vi "Swerve Math.vi"(0 "Gyro":dbl, 1 "FWD":dbl(slide) scale=-1.0..1.0, 2 "STR":dbl(slide) scale=-1.0..1.0, 3 "RCW":dbl(slide) scale=-1.0..1.0) -> (7 "Wheel Speeds":dbl[](array[numeric]), 9 "Wheel Angles":dbl[](array[numeric]))   [LabVIEW 2023]
uses:
  Framework/Robot Global Data.vi
panel:
  in  "Gyro Working":bool=TRUE
  out "STR(Field)":dbl
  out "FWD(Field)":dbl
  out "MAX(before normalized)":dbl
  out "WA 4":dbl
  out "WA 3":dbl
  out "WA 2":dbl
  out "WA 1":dbl
  out "WS 4":dbl
  out "WS 3":dbl
  out "WS 2":dbl
  out "WS 1":dbl
  out "D":dbl
  out "C":dbl
  out "B":dbl
  out "A":dbl
  in  "Width(Left to Right)":dbl=20.0
  in  "Length(Front to Back)":dbl=28.0
  # "From the Center of the Wheels"
  # "Forward/Back"
  # "Left/Right"
  # "Rotation(Clockwise)"
  # "Units are irrelevant"
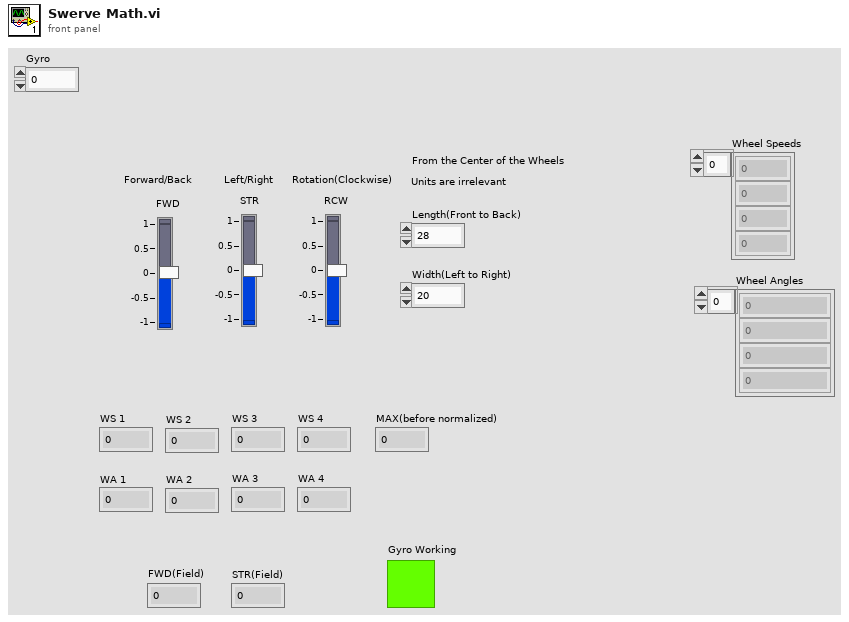
[diagram p1: front panel]
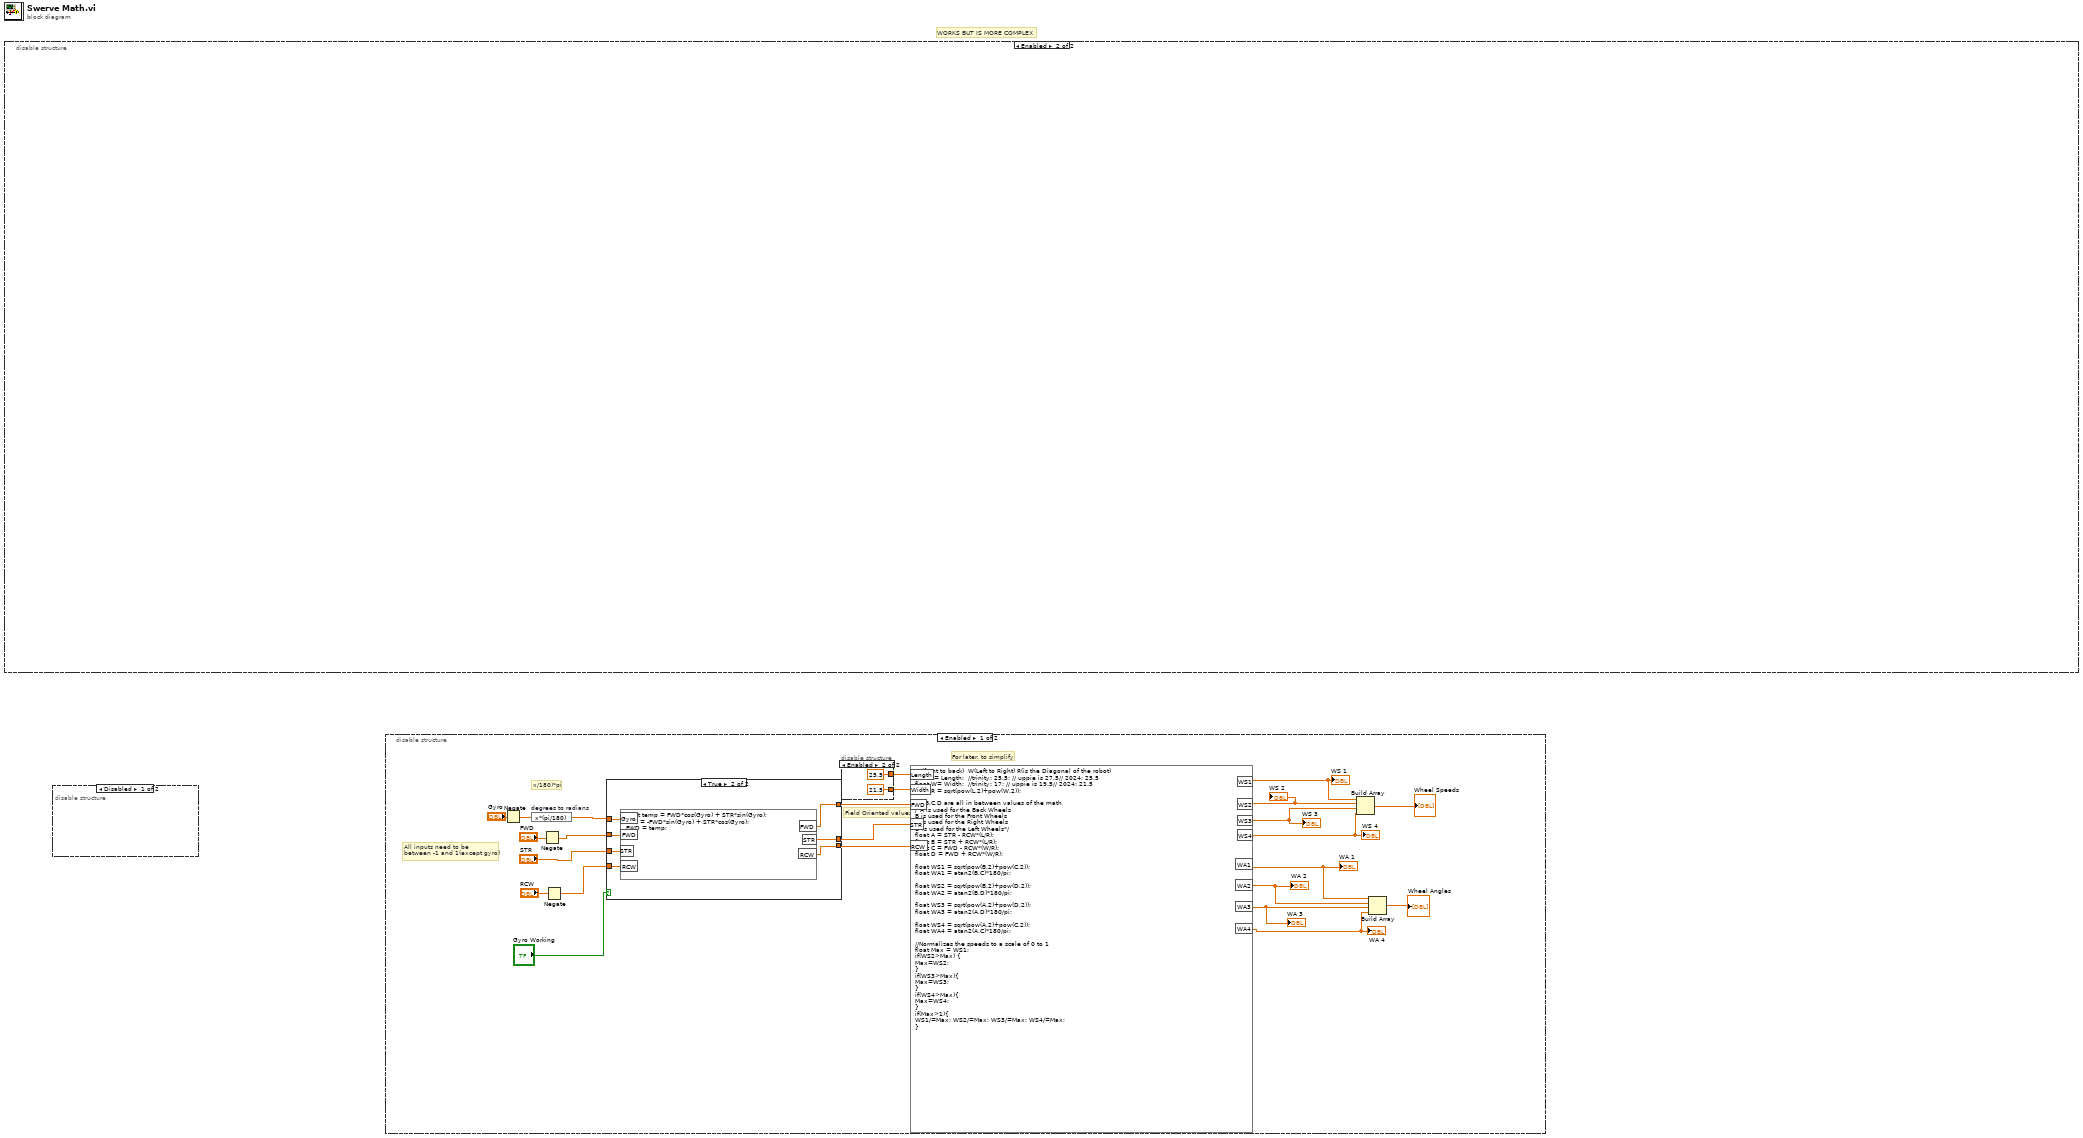
[diagram p0: block diagram]
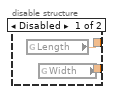
[diagram p3: hidden frame]
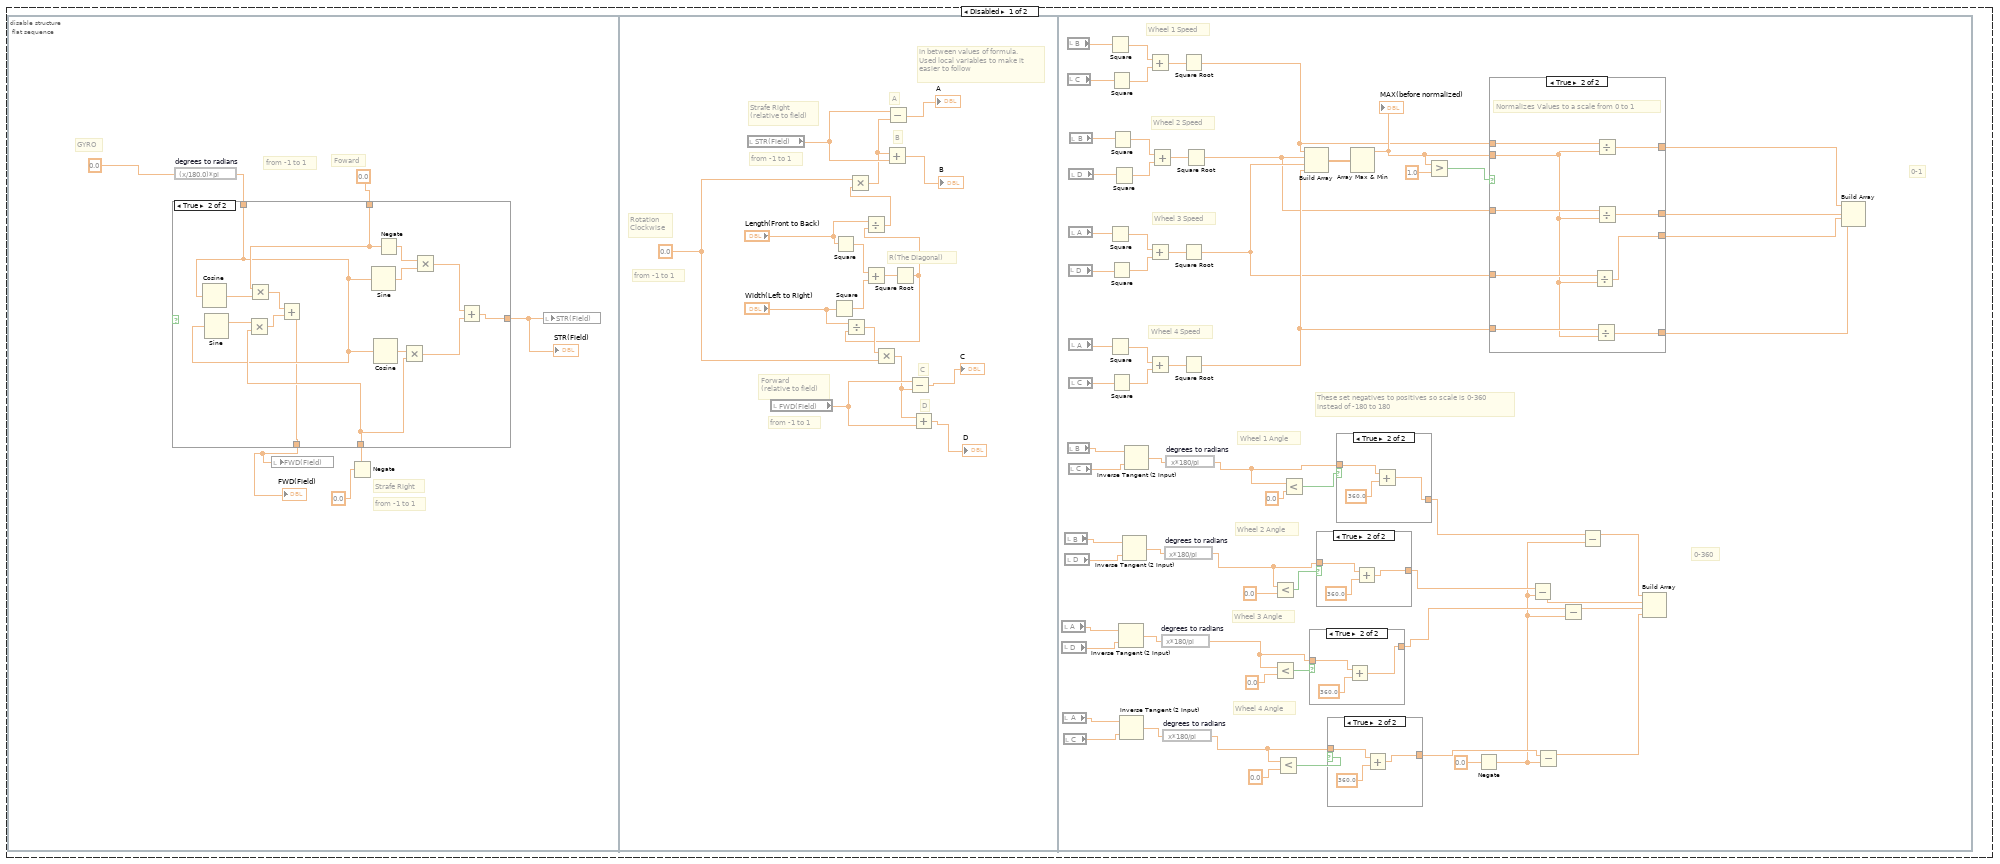
[diagram p6: hidden frame]
diagram:
  # "WORKS BUT IS MORE COMPLEX"
  n1 = disable-structure shown="Enabled" {
    frame Disabled {
      n2 = flat-sequence {
        frame #0 {
          # "GYRO"
          # "from -1 to 1"
          # "from -1 to 1"
          # "Strafe Right"
          # "Foward"
          n3 = expression code="(x/180.0)*pi" "degrees to radians"(0.0) -> (w5:dbl)
          n4 = Negate(x=0.0) -> (-x=w4:dbl)
          n5 = case shown="True" {
            selector: _ -> [_ _]
            tunnel: w4 -> [w9 w14]
            tunnel: 0.0 ("FWD") -> [w8 w13]
            tunnel: [w9 w12] -> w7
            tunnel: w5 -> [_ w11]
            tunnel: [w8 w10] -> w6
            frame False {
            }
            frame True {
              n6 = Cosine(x=w11) -> (cos(x)=w15:dbl)
              n7 = Sine(x=w11) -> (sin(x)=w16:dbl)
              n8 = Multiply(x=w16, y=w14) -> (x*y=w17:dbl)
              n9 = Multiply(x=w13, y=w15) -> (x*y=w18:dbl)
              n10 = Add(x=w18, y=w17) -> (x+y=w10:dbl)
              n11 = Sine(x=w11) -> (sin(x)=w23:dbl)
              n12 = Cosine(x=w11) -> (cos(x)=w22:dbl)
              n13 = Negate(x=w13) -> (-x=w21:dbl)
              n14 = Multiply(x=w22, y=w14) -> (x*y=w20:dbl)
              n15 = Multiply(x=w21, y=w23) -> (x*y=w19:dbl)
              n16 = Add(x=w19, y=w20) -> (x+y=w12:dbl)
            }
          }
          "STR(Field)" <- w7
          "FWD(Field)" <- w6
          n17 = local write "FWD(Field)"(w6) -> ()
          n18 = local write "STR(Field)"(w7) -> ()
        }
        frame #1 {
          w24 = 0.0 ("x")
          # "from -1 to 1"
          # "from -1 to 1"
          # "from -1 to 1"
          # "in between values of formula.\nUsed local variables to make it\neasier to follow"
          # "Rotation\nClockwise"
          # "Forward\n(relative to field)"
          # "Strafe Right\n(relative to field)"
          # "D"
          # "C"
          # "B"
          # "A"
          # "R(The Diagonal)"
          n19 = local read "STR(Field)"() -> (w40:dbl)
          n20 = local read "FWD(Field)"() -> (w39:dbl)
          n21 = Square(x="Width(Left to Right)") -> (x^2=w27:dbl)
          n22 = Square(x="Length(Front to Back)") -> (x^2=w26:dbl)
          n23 = Add(x=w26, y=w27) -> (x+y=w25:dbl)
          n24 = Square Root(x=w25) -> (sqrt(x)=w29:dbl)
          n25 = Divide(x="Width(Left to Right)", y=w29) -> (x/y=w32:dbl)
          n26 = Divide(x="Length(Front to Back)", y=w29) -> (x/y=w31:dbl)
          n27 = Multiply(x=w24, y=w31) -> (x*y=w33:dbl)
          n28 = Multiply(x=w32, y=w24) -> (x*y=w34:dbl)
          n29 = Add(x=w33, y=w40) -> (x+y=→"B":dbl)
          n30 = Subtract(x=w40, y=w33) -> (x-y=→"A":dbl)
          n31 = Subtract(x=w39, y=w34) -> (x-y=→"C":dbl)
          n32 = Add(x=w34, y=w39) -> (x+y=→"D":dbl)
        }
        frame #2 {
          # "0-360"
          # "0-1"
          # "These set negatives to positives so scale is 0-360\ninstead of -180 to 180"
          # "Wheel 4 Angle"
          # "Wheel 3 Angle"
          # "Wheel 2 Angle"
          # "Wheel 1 Angle"
          # "Wheel 4 Speed"
          # "Wheel 3 Speed"
          # "Wheel 2 Speed"
          # "Wheel 1 Speed"
          n33 = local read "A"() -> (w82:dbl)
          n34 = local read "D"() -> (w83:dbl)
          n35 = local read "A"() -> (w84:dbl)
          n36 = local read "C"() -> (w85:dbl)
          n37 = local read "B"() -> (w80:dbl)
          n38 = local read "D"() -> (w81:dbl)
          n39 = local read "B"() -> (w57:dbl)
          n40 = local read "C"() -> (w56:dbl)
          n41 = local read "B"() -> (w78:dbl)
          n42 = local read "D"() -> (w67:dbl)
          n43 = local read "C"() -> (w79:dbl)
          n44 = local read "D"() -> (w61:dbl)
          n45 = local read "A"() -> (w66:dbl)
          n46 = local read "A"() -> (w71:dbl)
          n47 = local read "C"() -> (w72:dbl)
          n48 = local read "B"() -> (w62:dbl)
          n49 = Square(x=w57) -> (x^2=w55:dbl)
          n50 = Square(x=w66) -> (x^2=w65:dbl)
          n51 = Square(x=w71) -> (x^2=w70:dbl)
          n52 = Square(x=w56) -> (x^2=w54:dbl)
          n53 = Square(x=w67) -> (x^2=w64:dbl)
          n54 = Square(x=w72) -> (x^2=w69:dbl)
          n55 = Square(x=w62) -> (x^2=w60:dbl)
          n56 = Square(x=w61) -> (x^2=w59:dbl)
          n57 = Inverse Tangent (2 Input)(1:w83, 2:w82) -> (0:w100:dbl)
          n58 = Inverse Tangent (2 Input)(1:w85, 2:w84) -> (0:w102:dbl)
          n59 = Inverse Tangent (2 Input)(1:w81, 2:w80) -> (0:w98:dbl)
          n60 = Inverse Tangent (2 Input)(1:w79, 2:w78) -> (0:w96:dbl)
          n61 = Add(x=w55, y=w54) -> (x+y=w53:dbl)
          n62 = Add(x=w65, y=w64) -> (x+y=w63:dbl)
          n63 = Add(x=w70, y=w69) -> (x+y=w68:dbl)
          n64 = Add(x=w60, y=w59) -> (x+y=w58:dbl)
          n65 = expression code="x*180/pi" "degrees to radians"(w100) -> (w101:dbl)
          n66 = expression code="x*180/pi" "degrees to radians"(w102) -> (w103:dbl)
          n67 = expression code="x*180/pi" "degrees to radians"(w98) -> (w99:dbl)
          n68 = expression code="x*180/pi" "degrees to radians"(w96) -> (w97:dbl)
          n69 = Square Root(x=w53) -> (sqrt(x)=w75:dbl)
          n70 = Square Root(x=w63) -> (sqrt(x)=w76:dbl)
          n71 = Square Root(x=w68) -> (sqrt(x)=w77:dbl)
          n72 = Square Root(x=w58) -> (sqrt(x)=w74:dbl)
          n73 = Less?(x=w99, y=0.0) -> (x < y?=w89:bool)
          n74 = Less?(x=w101, y=0.0) -> (x < y?=w88:bool)
          n75 = Less?(x=w103, y=0.0) -> (x < y?=w87:bool)
          n76 = Less?(x=w97, y=0.0) -> (x < y?=w86:bool)
          n77 = Build Array(w75, w74, w76, w77) -> (w73:dbl[])
          n78 = case shown="True" w88 {
            tunnel: w101 -> [w124 w126]
            tunnel: [w124 w125] -> w105
            frame False {
            }
            frame True {
              n79 = Add(x=w126, y=360.0) -> (x+y=w125:dbl)
            }
          }
          n80 = case shown="True" w89 {
            tunnel: w99 -> [w120 w122]
            tunnel: [w120 w121] -> w104
            frame False {
            }
            frame True {
              n81 = Add(x=w122, y=360.0) -> (x+y=w121:dbl)
            }
          }
          n82 = case shown="True" w87 {
            tunnel: w103 -> [w128 w130]
            tunnel: [w128 w129] -> w106
            frame False {
            }
            frame True {
              n83 = Add(x=w130, y=360.0) -> (x+y=w129:dbl)
            }
          }
          n84 = case shown="True" w86 {
            tunnel: w97 -> [w132 w134]
            tunnel: [w132 w133] -> w44
            frame False {
            }
            frame True {
              n85 = Add(x=w134, y=360.0) -> (x+y=w133:dbl)
            }
          }
          n86 = Array Max & Min(array=w73) -> (max value=w90:dbl)  [unwired: 3 out]
          "MAX(before normalized)" <- w90
          n87 = Greater?(x=w90, y=1.0) -> (0:w91:bool)
          n88 = Negate(x=0.0) -> (-x=w45:dbl)
          n89 = case shown="True" w91 {
            tunnel: w74 -> [w109 w119]
            tunnel: w75 -> [w110 w118]
            tunnel: w76 -> [w108 w117]
            tunnel: w77 -> [w107 w116]
            tunnel: w90 -> [_ w115]
            tunnel: [w110 w114] -> w92
            tunnel: [w109 w113] -> w93
            tunnel: [w108 w112] -> w94
            tunnel: [w107 w111] -> w95
            frame False {
            }
            frame True {
              # "Normalizes Values to a scale from 0 to 1"
              n90 = Divide(x=w117, y=w115) -> (x/y=w112:dbl)
              n91 = Divide(x=w116, y=w115) -> (x/y=w111:dbl)
              n92 = Divide(x=w118, y=w115) -> (x/y=w114:dbl)
              n93 = Divide(x=w119, y=w115) -> (x/y=w113:dbl)
            }
          }
          n94 = Subtract(x=w104, y=w45) -> (x-y=w42:dbl)
          n95 = Subtract(x=w106, y=w45) -> (x-y=w46:dbl)
          n96 = Subtract(x=w105, y=w45) -> (x-y=w43:dbl)
          n97 = Subtract(x=w44, y=w45) -> (x-y=w47:dbl)
          n98 = Build Array(w47, w42, w43, w46) -> ()  [unwired: 1 out]
          n99 = Build Array(w92, w93, w94, w95) -> ()  [unwired: 1 out]
        }
      }
    }
    frame Enabled {
    }
  }
  n100 = disable-structure shown="Disabled" {
    frame Disabled {
    }
    frame Enabled {
    }
  }
  n101 = disable-structure shown="Enabled" {
    frame Enabled {
      # "x/180)*pi"
      # "Field Oriented values"
      # "All inputs need to be\nbetween -1 and 1(except gyro)"
      # "For later, to simplify"
      n102 = Negate(x="Gyro") -> (-x=w136:dbl)
      n103 = expression code="x*(pi/180)" "degrees to radians"(w136) -> (w155:dbl)
      n104 = Negate(x="FWD") -> (-x=w142:dbl)
      n105 = Negate(x="RCW") -> (-x=w140:dbl)
      n106 = case shown="True" "Gyro Working" {
        tunnel: [w166 w173] -> w158
        tunnel: [w165 w172] -> w157
        tunnel: [w164 w171] -> w156
        tunnel: w155 -> [_ w170]
        tunnel: w142 -> [w166 w169]
        tunnel: w140 -> [w164 w168]
        tunnel: "STR" -> [w165 w167]
        frame False {
        }
        frame True {
          n107 = formula code="float temp = FWD*cos(Gyro) + STR*sin(Gyro); \nSTR = -FWD*sin(Gyro) + STR*cos(Gyro); \nFWD = temp;"("Gyro"=w170, "FWD"=w169, "STR"=w167, "RCW"=w168) -> ("FWD"=w173:dbl, "STR"=w172:dbl, "RCW"=w171:dbl)
        }
      }
      n108 = disable-structure shown="Enabled" {
        disable-tunnel: [w161 21.5 ("Width")] -> w139
        disable-tunnel: [w160 25.5 ("Length")] -> w138
        frame Disabled {
          n109 = global read "Robot Global Data.vi" "Length"() -> (w160:dbl)
          n110 = global read "Robot Global Data.vi" "Width"() -> (w161:dbl)
        }
        frame Enabled {
        }
      }
      n111 = formula code="//L(front to back)  W(Left to Right) R(is the Diagonal of the robot)\nfloat L= Length;  //trinity: 25.5; // uppie is 27.5// 2024: 25.5\nfloat W= Width;  //trinity: 17; // uppie is 19.5// 2024: 21.5\nfloat R = sqrt(pow(L,2)+pow(W,2));\n\n//A,B,C,D are all in between values of the math\n/*A is used for the Back Wheels\nB is used for the Front Wheels\nC is used for the Right Wheels\nD is used for the Left Wheels*/\nfloat A = STR - RCW*(L/R);\nfloat B = STR + RCW*(L/R);\nfloat C = FWD - RCW*(W/R);\nfloat D = FWD + RCW*(W/R); \n\nfloat WS1 = sqrt(pow(B,2)+pow(C,2));\nfloat WA1 = atan2(B,C)*180/pi;\n\nfloat WS2 = sqrt(pow(B,2)+pow(D,2));\nfloat WA2 = atan2(B,D)*180/pi;\n\nfloat WS3 = sqrt(pow(A,2)+pow(D,2));\nfloat WA3 = atan2(A,D)*180/pi;\n\nfloat WS4 = sqrt(pow(A,2)+pow(C,2));\nfloat WA4 = atan2(A,C)*180/pi;\n\n//Normalizes the speeds to a scale of 0 to 1\nfloat Max = WS1; \nif(WS2>Max) {\nMax=WS2; \n}\nif(WS3>Max){\nMax=WS3; \n}\nif(WS4>Max){\nMax=WS4; \n}\nif(Max>1){\nWS1/=Max; WS2/=Max; WS3/=Max; WS4/=Max;\n}"("FWD"=w158, "STR"=w157, "RCW"=w156, "Length"=w138, "Width"=w139) -> ("WS1"=w150:dbl, "WS2"=w147:dbl, "WS3"=w149:dbl, "WS4"=w148:dbl, "WA1"=w152:dbl, "WA3"=w153:dbl, "WA4"=w154:dbl, "WA2"=w159:dbl)
      "WA 1" <- w152
      "WA 2" <- w159
      "WA 3" <- w153
      "WA 4" <- w154
      "WS 1" <- w150
      "WS 2" <- w147
      "WS 3" <- w149
      "WS 4" <- w148
      n112 = Build Array(w150, w147, w149, w148) -> (→"Wheel Speeds":dbl[])
      n113 = Build Array(w152, w159, w153, w154) -> (→"Wheel Angles":dbl[])
    }
    frame Disabled {
    }
  }
